vi "Write Air Temperature Feedback.vi"(8 "error in (no error)":errorcluster, 10 "Temperature Feedback":dbl format="%#_13g", 11 "ThermotronDriver in":refnum<class "ThermotronDriver.lvclass">) -> (0 "error out":errorcluster, 3 "ThermotronDriver out":refnum<class "ThermotronDriver.lvclass">)   [LabVIEW 2023, in "ThermotronDriver.lvlib" / "ThermotronDriver.lvclass"]
uses:
  ThermotronDriver.lvclass
  ThermotronDriver.lvclass/ThermotronDriver.ctl
  <vilib>/ADAS Replay HIL/Channels/Tag Wrapper/Tag Wrapper.lvlib
  <vilib>/ADAS Replay HIL/Channels/Tag Wrapper/Polymorphic/Write Channel (Double).vi
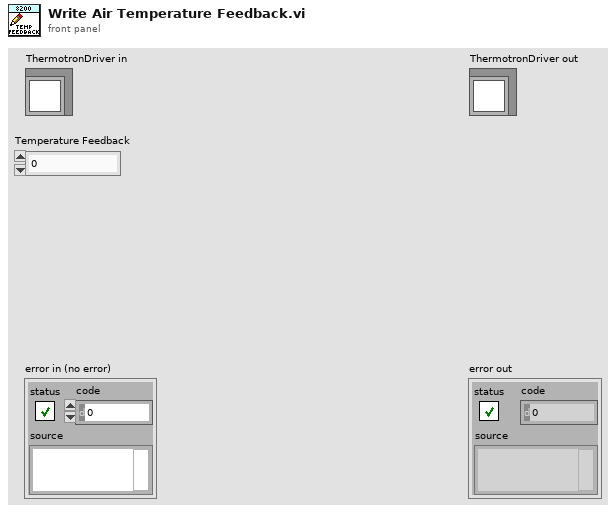
[diagram p1: front panel]
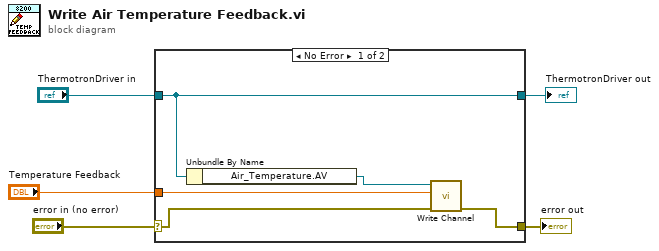
[diagram p0: block diagram]
diagram:
  n1 = case shown="No Error" "error in (no error)" {
    selector: "error in (no error)" -> [w10 w12]
    tunnel: [w9 w12] -> w4
    tunnel: [w8 w11] -> w2
    tunnel: "ThermotronDriver in" -> [w8 w11]
    tunnel: "Temperature Feedback" -> [w6 _]
    frame No Error {
      n2 = Unbundle By Name(w8) -> ("Air_Temperature.AV"=w7:refnum<k21>)
      n3 = call-poly <vilib>:"Write Channel.vi"("error in"=w10, "Value to Write"=w6, "ADAS HIL Channel in"=w7) -> ("error out"=w9:errorcluster)  [unwired: 6 in, 2 out]
    }
    frame Error {
    }
  }
  "error out" <- w4
  "ThermotronDriver out" <- w2
